vi "Write Alice Enq.vi"(8 "error in (no error)":errorcluster, 10 "Actor Framework:Message Enqueuer":refnum<class "Message Enqueuer.lvclass">, 11 "Bob in":refnum<class "Bob.lvclass">) -> (0 "error out":errorcluster, 3 "Bob out":refnum<class "Bob.lvclass">)   [LabVIEW 2014, in "Bob.lvlib" / "Bob.lvclass"]
uses:
  Bob.lvclass
  <vilib>/ActorFramework/Message Enqueuer/Message Enqueuer.lvclass
  Bob.lvclass/Bob.ctl
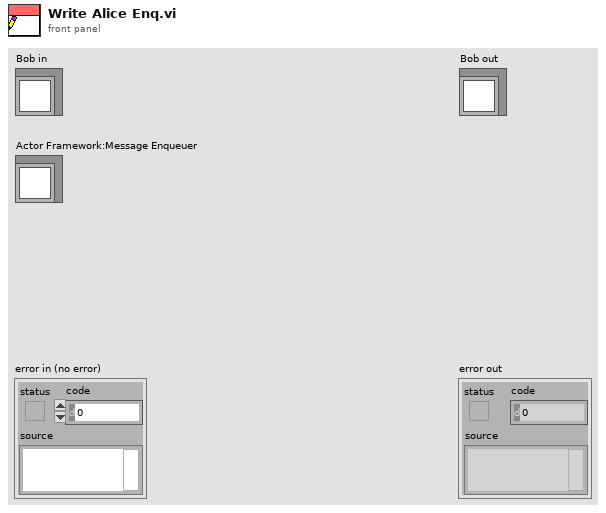
[diagram p1: front panel]
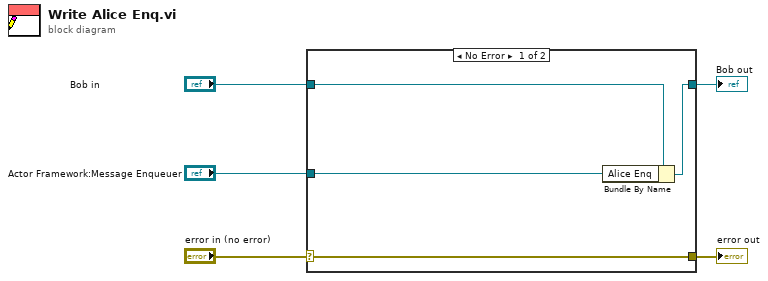
[diagram p0: block diagram]
diagram:
  n1 = case shown="No Error" "error in (no error)" {
    selector: "error in (no error)" -> [w9 w10]
    tunnel: [w9 w10] -> w4
    tunnel: [w7 w11] -> w2
    tunnel: "Bob in" -> [w8 w11]
    tunnel: "Actor Framework:Message Enqueuer" -> [w6 _]
    frame No Error {
      n2 = Bundle By Name(cluster=w8, "Alice Enq"=w6) -> (w7:refnum<class "Bob.lvclass">)
    }
    frame Error {
    }
  }
  "error out" <- w4
  "Bob out" <- w2
